vi "4155C Config Sampling Measurements.vi"(1 "Standby":T1, 2 "Sampling interval":dbl min=0.0 max=100000000000.0 format="%.6f", 4 "Sample time":dbl min=0.0 max=100000000000.0 format="%.2f", 5 "Display on/off":bool, 6 "Timings":T2={"integration time"=0, "Short/Long integration time"=0.00064, "hold time (sec)"=0.0, "delay time (sec)"=0.0, "Step Time (0 disables)"=0.0, "sweep method"=0, "Pulse period"=0.005, "Base voltage"=0.0, "Pulse width"=0.0005} {"Pulse width" min=0.0005 max=0.1 step=0.0001 format="%.4f"; "Base voltage" min=-100.0 max=100.0 format="%^.4e"; "Pulse period" min=0.005 max=1.0 step=0.0001 format="%.4f"; "sweep method" items=["Continuous", "Pulsed"]; "Step Time (0 disables)" format="%.2f"; "delay time (sec)" min=0.0 format="%.4f"; "hold time (sec)" min=0.0 format="%.4f"; "Short/Long integration time" min=0.0 format="%^.0e"; "integration time" scale=0.0..2.0}, 7 "Num Points":i16=1 min=1 max=1001, 8 "error in (no error)":errorcluster, 9 "Drain Compliance":dbl format="%.2f", 10 "Gate Compliance":dbl format="%.2f", 11 "VISA session":refnum<visa-resource-name>) -> (0 "error out":errorcluster, 3 "dup VISA resource name":refnum<visa-resource-name>)   [LabVIEW 2016]
doc: "This VI configures the primary sweep source (VAR1) for a sweep mode measurement. \n* This VI does not perform error checking on MEASUREMENT MODE or UNIT TYPE of VAR1, therefore it is the application programmer's responsibility to make certain this VI is used in the proper mode."
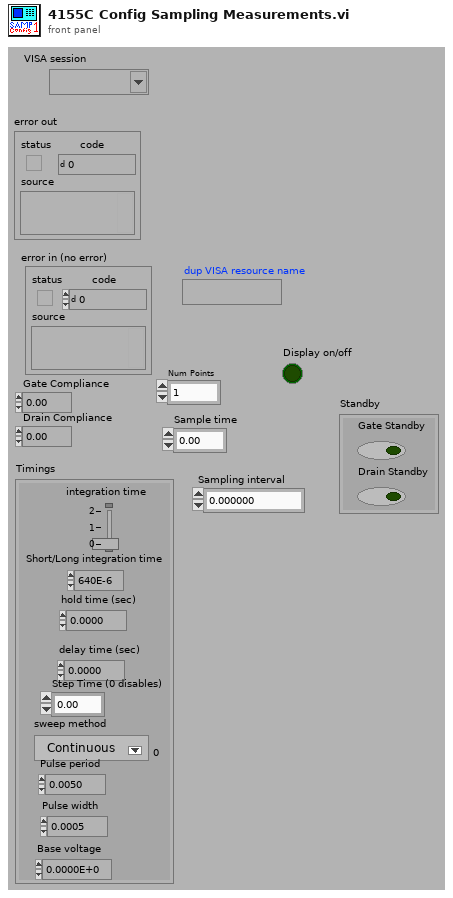
[diagram p1: front panel]
types:
  T1 = cluster{"Gate Standby":bool, "Drain Standby":bool}
  T2 = cluster{"integration time":u32, "Short/Long integration time":dbl, "hold time (sec)":dbl, "delay time (sec)":dbl, "Step Time (0 disables)":dbl, "sweep method":u16, "Pulse period":dbl, "Base voltage":dbl, "Pulse width":dbl}
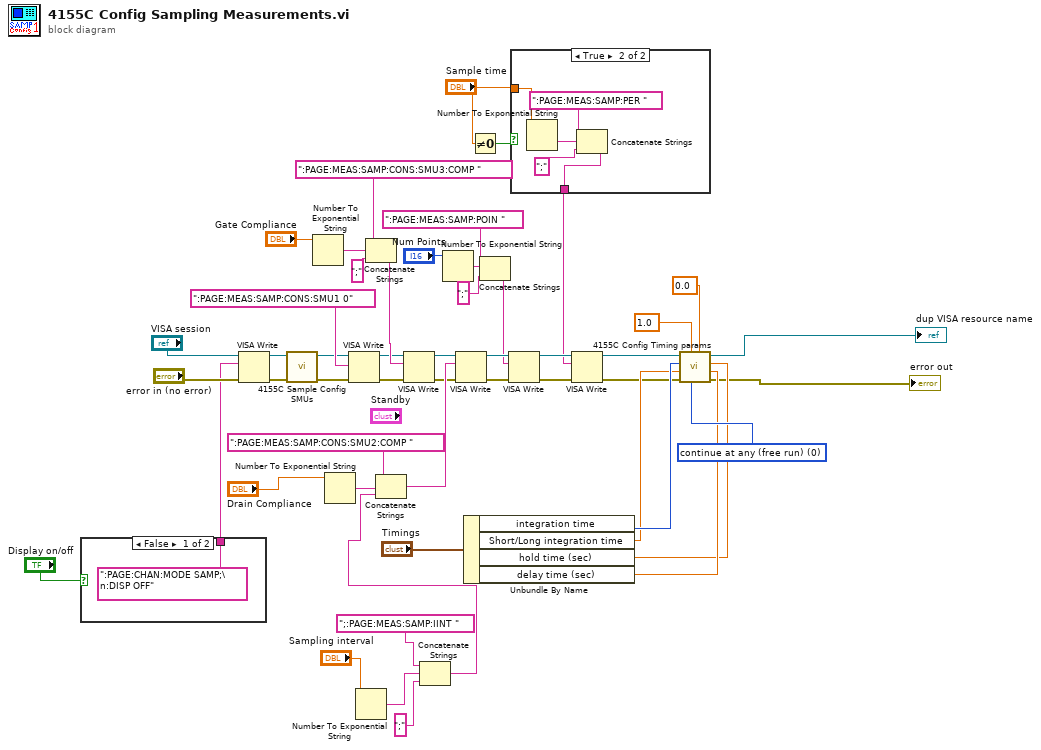
[diagram p0: block diagram]
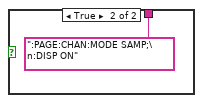
[diagram p2: hidden frame]
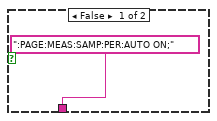
[diagram p3: hidden frame]
diagram:
  w36 = u8 0 items=["continue at any (free run)", "stop at any abnorm", "stop at compliance"] ("stop condition (free run:0)")
  n1 = case shown="False" "Display on/off" {
    tunnel: [":PAGE:CHAN:MODE SAMP;\n:DISP OFF" ("write buffer (\"\")") ":PAGE:CHAN:MODE SAMP;\n:DISP ON" ("write buffer (\"\")")] -> w6
    frame False {
    }
    frame True {
    }
  }
  n2 = VISA Write(VISA resource name="VISA session", write buffer=w6, error in (no error)="error in (no error)") -> (VISA resource name out=w25:refnum<visa-resource-name>, error out=w24:errorcluster)  [unwired: 1 out]
  n3 = call "4155C Sample Config SMUs.vi"("error in (no error)"=w24, "VISA resource name in"=w25) -> ("error out"=w23:errorcluster, "VISA Resource Name out"=w22:refnum<visa-resource-name>)  [unwired: 4 in]
  n4 = Number To Exponential String(number="Gate Compliance") -> (E-format string=w44:string)  [unwired: 3 in]
  n5 = Number To Exponential String(number="Drain Compliance") -> (E-format string=w46:string)  [unwired: 3 in]
  n6 = VISA Write(VISA resource name=w22, write buffer=":PAGE:MEAS:SAMP:CONS:SMU1 0" ("write buffer (\"\")"), error in (no error)=w23) -> (VISA resource name out=w42:refnum<visa-resource-name>, error out=w41:errorcluster)  [unwired: 1 out]
  n7 = Number To Exponential String(number="Sampling interval") -> (E-format string=w5:string)  [unwired: 3 in]
  n8 = Concatenate Strings(":PAGE:MEAS:SAMP:CONS:SMU3:COMP ", w44, ";" ("Substring")) -> (w45:string)
  n9 = VISA Write(VISA resource name=w42, write buffer=w45, error in (no error)=w41) -> (VISA resource name out=w39:refnum<visa-resource-name>, error out=w38:errorcluster)  [unwired: 1 out]
  n10 = Concatenate Strings(";:PAGE:MEAS:SAMP:IINT ", w5, ";" ("Substring")) -> (w2:string)
  n11 = Concatenate Strings(":PAGE:MEAS:SAMP:CONS:SMU2:COMP ", w46, w2) -> (w49:string)
  n12 = Number To Exponential String(number="Num Points") -> (E-format string=w20:string)  [unwired: 3 in]
  n13 = VISA Write(VISA resource name=w39, write buffer=w49, error in (no error)=w38) -> (VISA resource name out=w50:refnum<visa-resource-name>, error out=w51:errorcluster)  [unwired: 1 out]
  n14 = Unbundle By Name("Timings") -> ("integration time"=w33:u32, "Short/Long integration time"=w28:dbl, "hold time (sec)"=w34:dbl, "delay time (sec)"=w35:dbl)
  n15 = Not Equal To 0?(x="Sample time") -> (x != 0?=w13:bool)
  n16 = Concatenate Strings(":PAGE:MEAS:SAMP:POIN " ("write buffer (\"\")"), w20, ";" ("Substring")) -> (w15:string)
  n17 = VISA Write(VISA resource name=w50, write buffer=w15, error in (no error)=w51) -> (VISA resource name out=w12:refnum<visa-resource-name>, error out=w11:errorcluster)  [unwired: 1 out]
  n18 = case shown="True" w13 {
    tunnel: "Sample time" -> [_ w58]
    tunnel: [":PAGE:MEAS:SAMP:PER:AUTO ON;" w55] -> w8
    frame False {
    }
    frame True {
      n19 = Number To Exponential String(number=w58) -> (E-format string=w59:string)  [unwired: 3 in]
      n20 = Concatenate Strings(":PAGE:MEAS:SAMP:PER " ("Substring"), w59, ";" ("Substring")) -> (w55:string)
    }
  }
  n21 = VISA Write(VISA resource name=w12, write buffer=w8, error in (no error)=w11) -> (VISA resource name out=w9:refnum<visa-resource-name>, error out=w10:errorcluster)  [unwired: 1 out]
  n22 = call "4155C Config Timing params.vi"("delay time (sec)"=w35, "hold time (sec)"=w34, "Step Time (0 disables)"=0.0, "stop condition (free run:0)"=w36, "wait time parameter"=1.0, "error in (no error)"=w10, "Short/Long integration time"=w28, "integration time"=w33, "VISA session"=w9) -> ("error out"=→"error out":errorcluster, "dup VISA resource name"=→"dup VISA resource name":refnum<visa-resource-name>)  [unwired: 1 in]
